vi "Process Data.vi"(8 "error in (no error)":errorcluster, 10 "AbstractData in":refnum<class "AbstractData.lvclass">, 11 "AbstractProcessor1D in":refnum<class "AbstractProcessor1D.lvclass">) -> (0 "error out":errorcluster, 2 "AbstractData out":refnum<class "AbstractData.lvclass">, 3 "AbstractProcessor1D out":refnum<class "AbstractProcessor1D.lvclass">)   [LabVIEW 2014, in "AbstractProcessor1D.lvclass"]
uses:
  AbstractProcessor1D.lvclass
  Model/Data/AbstractData/AbstractData.lvclass
  Model/Data/Data1D/Data1D.lvclass
  Data1D Cluster.ctl
  Interfaces/Observable Actor/Observable Actor.lvclass
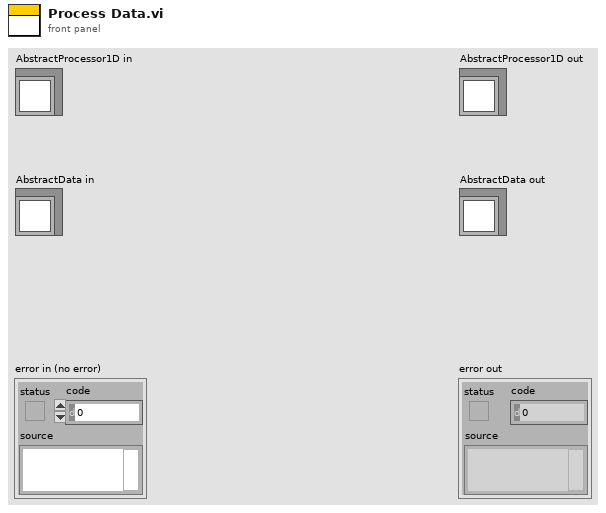
[diagram p1: front panel]
types:
  T1 = typedef "AbstractProcessor1D.lvclass/Data1D Cluster.ctl" = cluster{"in":refnum<class "Data1D.lvclass">, "out":refnum<class "Data1D.lvclass">}
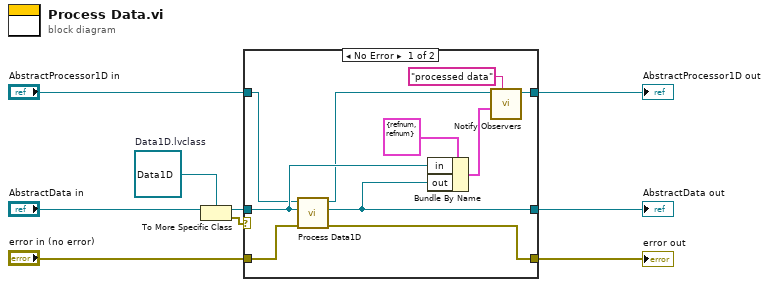
[diagram p0: block diagram]
diagram:
  w9 = refnum<class "Data1D.lvclass"> refnum  # Data1D.lvclass
  n1 = To More Specific Class(target class=w9, reference="AbstractData in") -> (specific class reference=w8:refnum<class "Data1D.lvclass">, error out=w2:errorcluster)  [unwired: 1 in]
  n2 = case shown="No Error" w2 {
    tunnel: w8 -> [w17 w20]
    tunnel: "error in (no error)" -> [w19 w22]
    tunnel: [w18 w22] -> w5
    tunnel: "AbstractProcessor1D in" -> [w12 w21]
    tunnel: [w13 w21] -> w7
    tunnel: [w16 w20] -> w4
    frame No Error {
      n3 = call-dynamic "Process Data1D.vi"("error in (no error)"=w19, "Data1D in"=w17, "AbstractProcessor1D in"=w12) -> ("error out"=w18:errorcluster, "Data1D out"=w16:refnum<class "Data1D.lvclass">, "AbstractProcessor1D out"=w11:refnum<class "AbstractProcessor1D.lvclass">)  [unwired: 6 in]
      n4 = Bundle By Name(cluster=T1 {"in"=refnum, "out"=refnum} ("Cluster"), "in"=w17, "out"=w16) -> (w14:T1)
      n5 = call "Notify Observers.vi"("name"="processed data", "value"=w14, "Observable Actor in"=w11) -> ("Observable Actor out"=w13:refnum<class "AbstractProcessor1D.lvclass">)  [unwired: 7 in, 1 out]
    }
    frame Error {
    }
  }
  "error out" <- w5
  "AbstractProcessor1D out" <- w7
  "AbstractData out" <- w4
